vi "nirviMemWrite.vi"(1 "Data":u16, 2 "Address":u16) -> (0 "Failure":bool)   [LabVIEW 2017]
doc: "<B>LabVIEW no longer supports this VI. Use the Memory Write function configured for a memory item instead.</B>\n\nWrites to memory available on the FPGA. You can access the memory only as 16-bit words. There are 16 KB of memory available, organized as 8 K x 16 bits. Use the Memory Write VI in conjunction with the Memory Read VI.\n\nIf you use the Memory Write VI in a single-cycle Timed Loop, you cannot use the VI anywhere else on the block diagram."
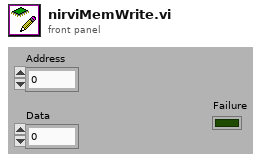
[diagram p1: front panel]
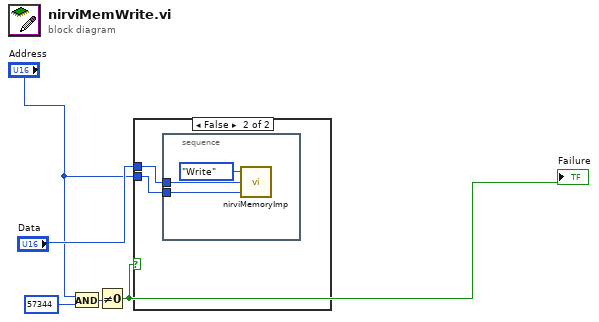
[diagram p0: block diagram]
diagram:
  n1 = And(x="Address", y=u16 57344) -> (x .and. y?=w5:u16)
  n2 = Not Equal To 0?(x=w5) -> (x != 0?=w1:bool)
  "Failure" <- w1
  n3 = case shown="False" w1 {
    tunnel: "Data" -> [_ w7]
    tunnel: "Address" -> [_ w6]
    frame True {
    }
    frame False {
      n4 = stacked-sequence {
        tunnel: w7 -> [w9]
        tunnel: w6 -> [w8]
        frame #0 {
          n5 = call <vilib>:"nirviMemoryImp.vi"("Address"=w8, "Data"=w9, "Enum"=enum16{"Read", "Write"}."Write") -> ()  [unwired: 1 out]
        }
      }
    }
  }
